vi "SCPI Configure Program.vi"(8 "error in (no error)":errorcluster, 9 "Steps":u16, 10 "Cycles":u16, 11 "VISA resource name":refnum<visa-resource-name>) -> (0 "error out":errorcluster, 3 "VISA resource name out":refnum<visa-resource-name>)   [LabVIEW 2021, in "BK Precision 169XB.lvlib"]
doc: "Configures over current protection (OCP). Specify the output current limit value and the behavior of the power supply when the output current is greater than or equal to that value."
uses:
  BK Precision 169XB.lvlib
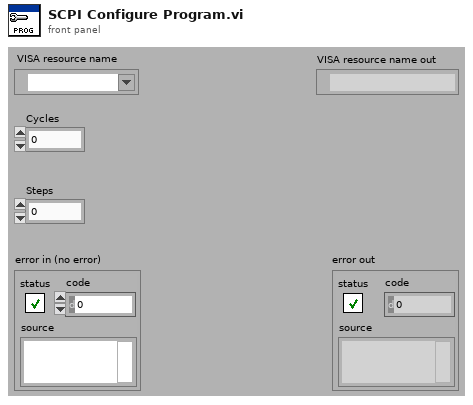
[diagram p1: front panel]
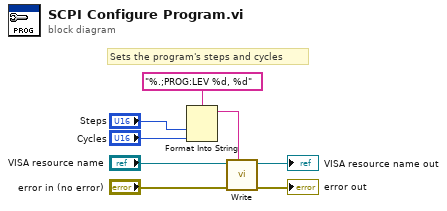
[diagram p0: block diagram]
diagram:
  # "Sets the program's steps and cycles"
  n1 = Format Into String(format string="%.;PROG:LEV %d, %d", "Steps", "Cycles") -> (resulting string=w8:string)  [unwired: 2 in, 1 out]
  n2 = call "Write.vi"("Input String"=w8, "error in (no error)"="error in (no error)", "VISA resource name"="VISA resource name") -> ("error out"=→"error out":errorcluster, "VISA resource name out"=→"VISA resource name out":refnum<visa-resource-name>)  [unwired: 6 in, 1 out]
